vi "DriveAutoCommand.vi"(10 "RightDriveMagnatude":dbl, 11 "LeftDriveMagnatude":dbl) -> ()   [LabVIEW 2017, in "AutoDrive.lvclass"]
uses:
  AutoSubsystem/AutoDrive/AutoDrive.lvclass
  SubsystemData/DriveData/DriveCommand.ctl
  SubsystemData/DriveData/DriveData.lvclass
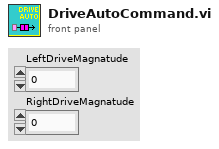
[diagram p1: front panel]
types:
  T1 = typedef "DriveData.lvclass/DriveCommand.ctl" = cluster{"RightDriveMagnatude":dbl, "LeftDriveMagnatude":dbl}
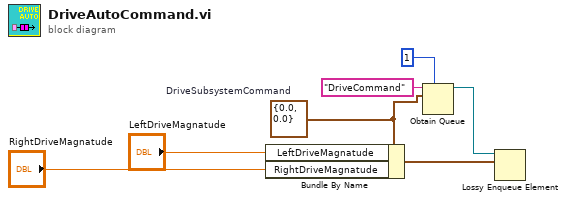
[diagram p0: block diagram]
diagram:
  w7 = T1 {"RightDriveMagnatude"=0.0, "LeftDriveMagnatude"=0.0}  # DriveSubsystemCommand
  n1 = Bundle By Name(cluster=w7, "LeftDriveMagnatude"="LeftDriveMagnatude", "RightDriveMagnatude"="RightDriveMagnatude") -> (w4:T1)
  n2 = Obtain Queue(max queue size (-1, unlimited)=1, name (unnamed)="DriveCommand", element data type=w7) -> (queue out=w3:refnum<queue>)  [unwired: 2 in, 2 out]
  n3 = Lossy Enqueue Element(queue=w3, element=w4) -> ()  [unwired: 1 in, 4 out]
